vi "Create_Trajectories.vi"(8 "error in":errorcluster caption="entrée d'erreur", 11 "Type of pattern":T1(ring)) -> (0 "error out":errorcluster caption="sortie d'erreur", 2 "Graphe XY":cluster{dbl[], dbl[]}(graph), 3 "Graphe":dbl[][](graph))   [LabVIEW 2026]
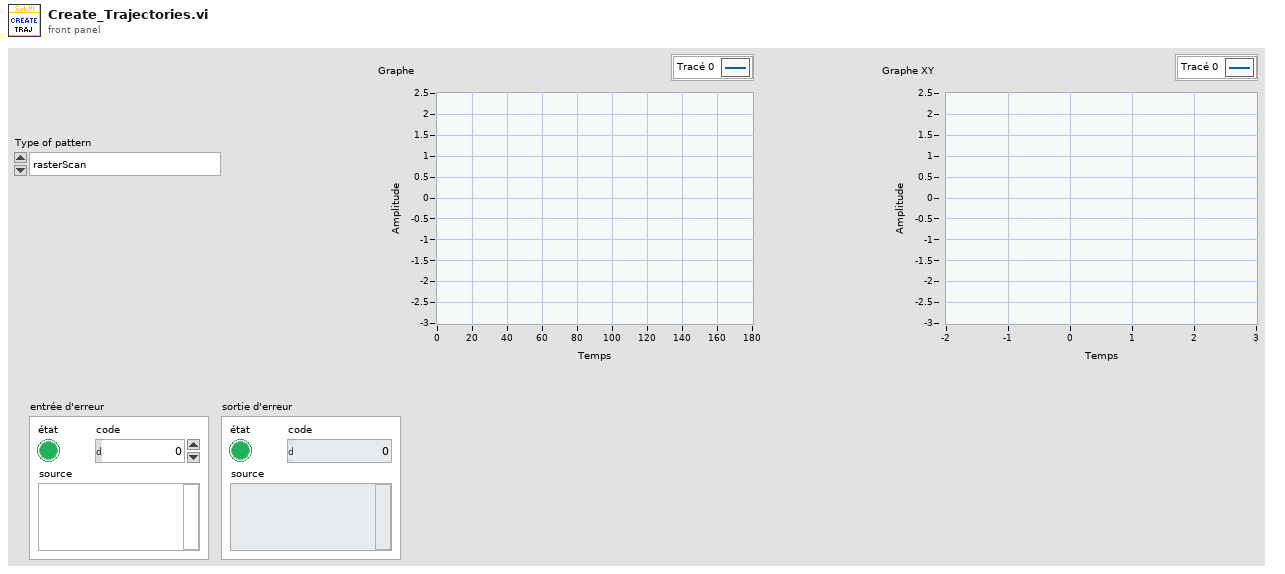
[diagram p1: front panel]
types:
  T1 = enum16{"rasterScan", "snakeMovement", "circularScan", "circularTIR", "spiralScan"}
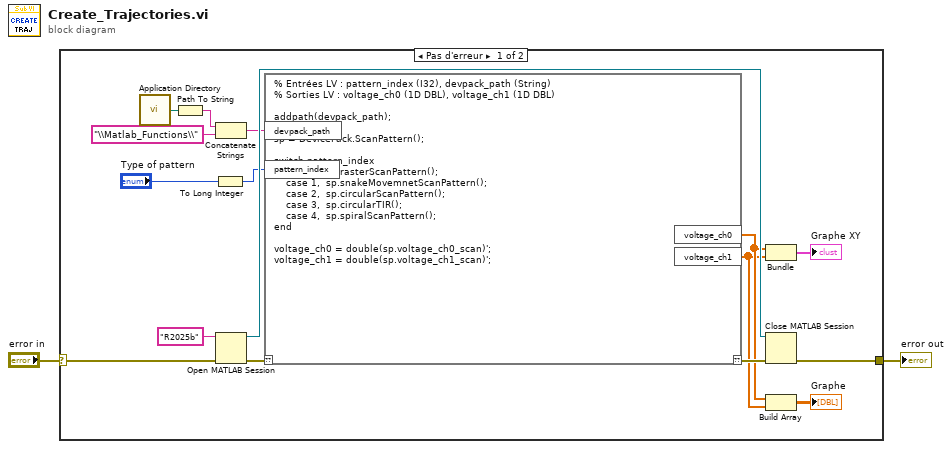
[diagram p0: block diagram]
diagram:
  n1 = case shown="Pas d'erreur" "error in" {
    selector: "error in" -> [w16 w19]
    tunnel: [w18 w19] -> w1
    frame No Error {
      n2 = call <vilib>:"Application Directory.vi"() -> ("Application Directory"=w11:path)
      n3 = Path To String(path=w11) -> (string=w13:string)
      n4 = To Long Integer(number="Type of pattern") -> (32bit integer=w8:i32)
      n5 = Concatenate Strings(w13, "\\Matlab_Functions\\" ("chaîne")) -> (w7:string)
      n6 = Open MATLAB Session(0:"R2025b" ("nom de version"), 3:w16) -> (8:w17:refnum<k37>, 11:w10:errorcluster)
      n7 = script code="% Entrées LV : pattern_index (I32), devpack_path (String)\n% Sorties LV : voltage_ch0 (1D DBL), voltage_ch1 (1D DBL)\n\naddpath(devpack_path);\n\nsp = DevicePack.ScanPattern();\n\nswitch pattern_index\n    case 0,  sp.rasterScanPattern();\n    case 1,  sp.snakeMovemnetScanPattern();\n    case 2,  sp.circularScanPattern();\n    case 3,  sp.circularTIR();\n    case 4,  sp.spiralScanPattern();\nend\n\nvoltage_ch0 = double(sp.voltage_ch0_scan)';\nvoltage_ch1 = double(sp.voltage_ch1_scan)';"("??"=w10, "pattern_index"=w8, "devpack_path"=w7) -> ("??"=w9:errorcluster, "voltage_ch0"=w5:dbl[], "voltage_ch1"=w4:dbl[])
      n8 = Bundle(w5, w4) -> (→"Graphe XY":cluster{dbl[], dbl[]})  [unwired: 1 in]
      n9 = Close MATLAB Session(0:w17, 3:w9) -> (11:w18:errorcluster)
      n10 = Build Array(w5, w4) -> (→"Graphe":dbl[][])
    }
    frame Error {
    }
  }
  "error out" <- w1
